vi "NewChicagoStylePepperoniPizza.vi"(8 "error in (no error)":errorcluster) -> (0 "error out":errorcluster, 3 "ChicagoStylePepperoniPizza":refnum<class "ChicagoStylePepperoniPizza.lvclass">)   [LabVIEW 2020, in "FactoryMethod.lvlib" / "PizzaFactoryMethod.lvlib" / "ChicagoStylePepperoniPizza.lvclass"]
uses:
  ChicagoStylePepperoniPizza.lvclass
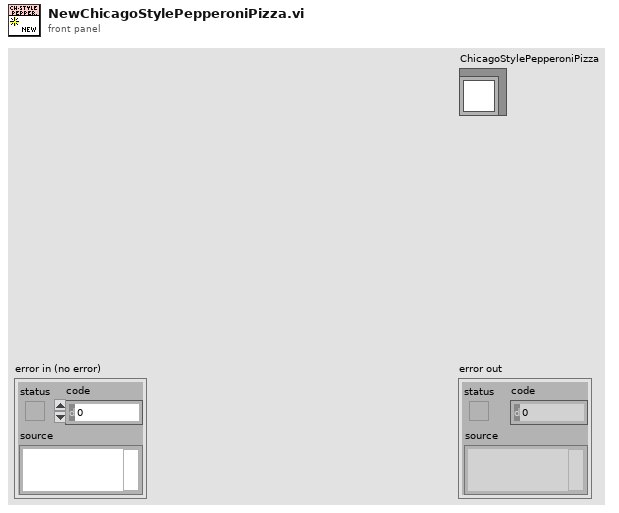
[diagram p1: front panel]
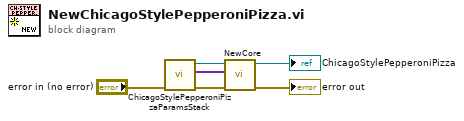
[diagram p0: block diagram]
diagram:
  n1 = call "ChicagoStylePepperoniPizzaParamsStack.vi"("error iN"="error in (no error)") -> ("error out"=w6:errorcluster, "HierarchyParams"=w5:variant[], "ChicagoStylePepperoniPizza"=w1:refnum<class "ChicagoStylePepperoniPizza.lvclass">)  [unwired: 8 in]
  n2 = call-dynamic "NewCore.vi"("error in (no error)"=w6, "ParamsArray"=w5, "ChicagoStylePepperoniPizza"=w1) -> ("error out"=→"error out":errorcluster, "ChicagoStylePepperoniPizza"=→"ChicagoStylePepperoniPizza":refnum<class "ChicagoStylePepperoniPizza.lvclass">)  [unwired: 7 in]
